vi "PSTR-Initialize Data.vi"(0 "PSTR Params":T1={"Stimulus"={"Ear"=enum."Right", "BW (oct)"=0.25, "Seed"=37, "Ramp (ms)"=5.0, "On time (ms)"=300.0, "Off time (ms)"=300.0, "Delay (ms)"=10000.0}, "FreqSeq"={"Min (kHz)"=4.0, "Max (kHz)"=64.0, "Step (oct)"=0.5}, "LevelSeq"={"Min (dB)"=0.0, "Max (dB)"=80.0, "Step (dB)"=20.0}, "Seq"={"Order"=enum."Sequential", "Averages"=20}, "Response"={"Grass gain"=10000.0, "Window (ms)"=0.0}, "Hidden"={"Sample rate (Hz)"=200000.0, "Nfft"=0, "save raw"=FALSE, "sep"=0.0, "Window"=enum."NONE"}, "RejThr"=0.0}) -> (8 "Data":T10, 15 "error out":errorcluster)   [LabVIEW 2020]
uses:
  Typedefs/PSTR-Data.ctl
  Typedefs/PSTR-Fit Parameters.ctl
  Typedefs/PSTR-Model Fit.ctl
  epl-vi-lib/Utility VIs/Math VIs/LinSpace (x0-dx-npts).vi
  epl-vi-lib/Utility VIs/Math VIs/LinSpace (start-stop-step).vi
  Utility VIs/Type Defs/Left-Right ring.ctl
  Typedefs/PSTR-Stimulus Params.ctl
  Typedefs/PSTR-FreqSeq Params.ctl
  Typedefs/PSTR-LevelSeq Params.ctl
  Typedefs/PSTR-SeqParams.ctl
  Typedefs/PSTR-Response Params.ctl
  Typedefs/PSTR-Hidden Params.ctl
  Typedefs/PSTR-Parameters.ctl
  Typedefs/PSTR-Window Shape.ctl
panel:
  # "NF x NL x 2 x Npts"
  # "NF x NL x Npts"
  # "NF x NL"
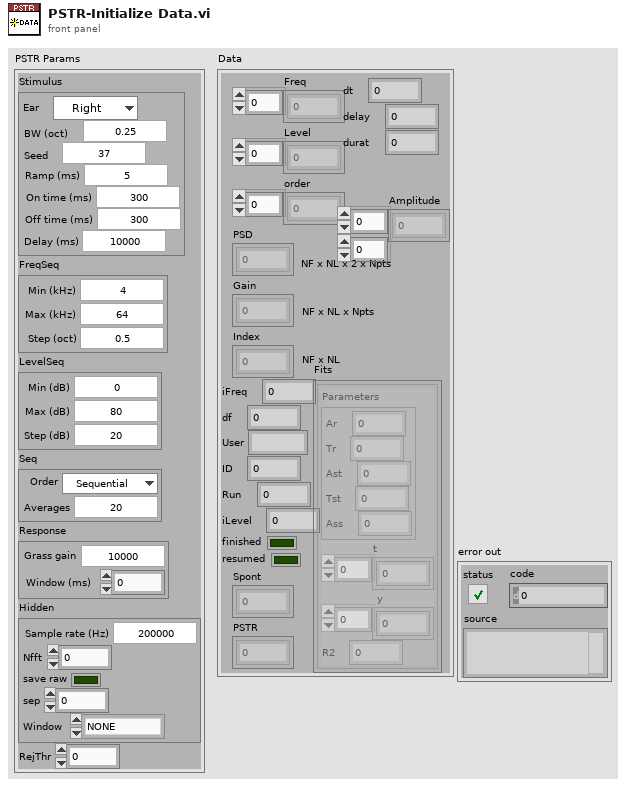
[diagram p1: front panel]
types:
  T1 = typedef "PSTR-Parameters.ctl" = cluster{"Stimulus":T2, "FreqSeq":T4, "LevelSeq":T5, "Seq":T6, "Response":T7, "Hidden":T8, "RejThr":dbl}
  T2 = typedef "PSTR-Stimulus Params.ctl" = cluster{"Ear":T3, "BW (oct)":dbl, "Seed":i32, "Ramp (ms)":dbl, "On time (ms)":dbl, "Off time (ms)":dbl, "Delay (ms)":dbl}
  T3 = typedef "Left-Right ring.ctl" = enum16{"Right", "Left"}
  T4 = typedef "PSTR-FreqSeq Params.ctl" = cluster{"Min (kHz)":dbl, "Max (kHz)":dbl, "Step (oct)":dbl}
  T5 = typedef "PSTR-LevelSeq Params.ctl" = cluster{"Min (dB)":dbl, "Max (dB)":dbl, "Step (dB)":dbl}
  T6 = typedef "PSTR-SeqParams.ctl" = cluster{"Order":enum16{"Sequential", "Random"}, "Averages":i32}
  T7 = typedef "PSTR-Response Params.ctl" = cluster{"Grass gain":dbl, "Window (ms)":dbl}
  T8 = typedef "PSTR-Hidden Params.ctl" = cluster{"Sample rate (Hz)":dbl, "Nfft":i32, "save raw":bool, "sep":dbl, "Window":T9}
  T9 = typedef "PSTR-Window Shape.ctl" = enum16{"NONE", "Hamming"}
  T10 = typedef "PSTR-Data.ctl" = cluster{"Freq":dbl[], "Level":dbl[], "order":i32[], "PSD":dbl[][][][], "Gain":dbl[][][], "Index":dbl[][], "iFreq":i32, "df":dbl, "User":string, "ID":i32, "Run":i32, "iLevel":i32, "finished":bool, "resumed":bool, "Spont":dbl[][], "PSTR":dbl[][][], "dt":dbl, "delay":dbl, "durat":dbl, "Fits":T11[][], "Amplitude":dbl[][]}
  T11 = typedef "PSTR-Model Fit.ctl" = cluster{"Parameters":T12, "t":dbl[], "y":dbl[], "R2":dbl}
  T12 = typedef "PSTR-Fit Parameters.ctl" = cluster{"Ar":dbl, "Tr":dbl, "Ast":dbl, "Tst":dbl, "Ass":dbl}
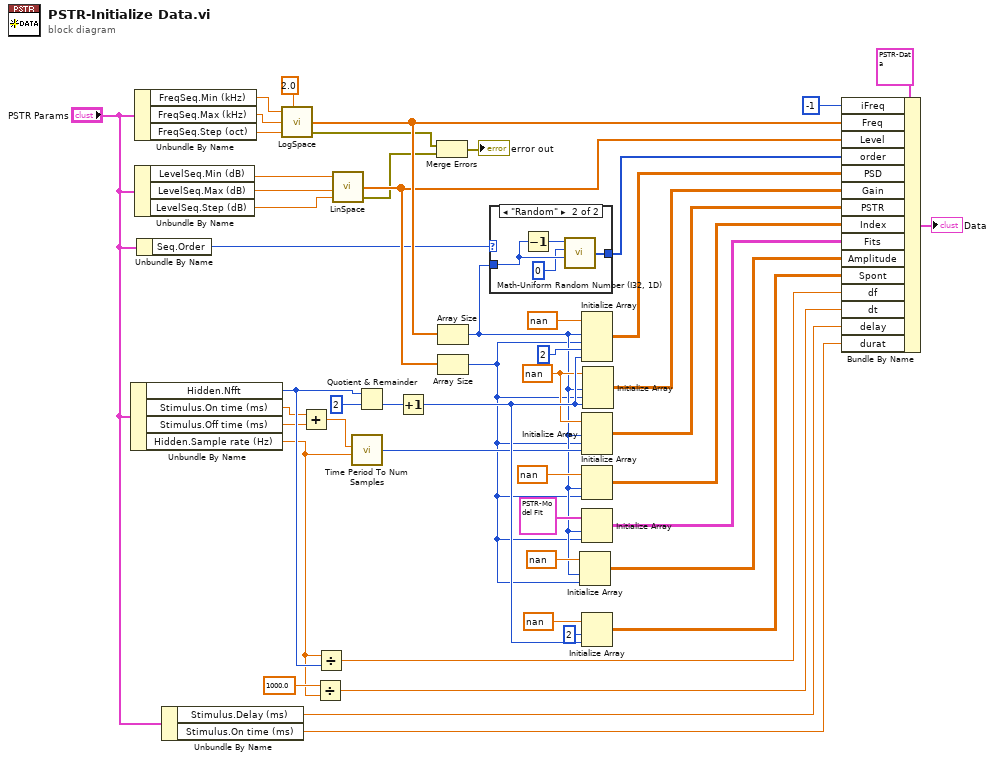
[diagram p0: block diagram]
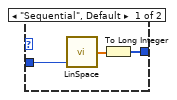
[diagram p2: hidden frame]
diagram:
  w10 = nan ("element")
  n1 = Unbundle By Name("PSTR Params") -> ("Hidden.Nfft"=w25:i32, "Stimulus.On time (ms)"=w14:dbl, "Stimulus.Off time (ms)"=w11:dbl, "Hidden.Sample rate (Hz)"=w13:dbl)
  n2 = Unbundle By Name("PSTR Params") -> ("FreqSeq.Min (kHz)"=w49:dbl, "FreqSeq.Max (kHz)"=w48:dbl, "FreqSeq.Step (oct)"=w47:dbl)
  n3 = Unbundle By Name("PSTR Params") -> ("LevelSeq.Min (dB)"=w42:dbl, "LevelSeq.Max (dB)"=w41:dbl, "LevelSeq.Step (dB)"=w40:dbl)
  n4 = Unbundle By Name("PSTR Params") -> ("Seq.Order"=w29:enum16{"Sequential", "Random"})
  n5 = Unbundle By Name("PSTR Params") -> ("Stimulus.Delay (ms)"=w8:dbl, "Stimulus.On time (ms)"=w7:dbl)
  n6 = call "LogSpace.vi"("Start"=w49, "Base"=2.0, "Stop"=w48, "Step"=w47) -> ("Array"=w38:dbl[], "error out"=w31:errorcluster)  [unwired: 2 in]
  n7 = Add(x=w14, y=w11) -> (x+y=w12:dbl)
  n8 = Divide(x=1000.0, y=w13) -> (x/y=w19:dbl)
  n9 = Divide(x=w13, y=w25) -> (x/y=w20:dbl)
  n10 = call-poly "LinSpace.vi"("Step"=w40, "Stop"=w41, "Start"=w42) -> ("error out"=w30:errorcluster, "Array"=w37:dbl[])  [unwired: 1 in]
  n11 = call "Time Period To Num Samples.vi"("Duration (ms)"=w12, "Sampling rate (Hz)"=w13) -> ("Samples"=w15:i32)  [unwired: 5 in]
  n12 = Quotient & Remainder(x=w25, y=2) -> (floor(x/y)=w26:i32)  [unwired: 1 out]
  n13 = Increment(x=w26) -> (x+1=w18:i32)
  n14 = Merge Errors(w31, w30) -> (→"error out":errorcluster)
  n15 = Array Size(array=w38) -> (size(s)=w3:i32)
  n16 = Array Size(array=w37) -> (size(s)=w2:i32)
  n17 = case shown="\"Random\"" w29 {
    tunnel: w3 -> [w52 w54]
    tunnel: [w50 w55] -> w28
    frame "Sequential", Default {
      n18 = call-poly "LinSpace.vi"("npts"=w52) -> ("Array"=w51:dbl[])  [unwired: 3 in, 1 out]
      n19 = To Long Integer(number=w51) -> (32bit integer=w50:i32[])
    }
    frame "Random" {
      n20 = Decrement(x=w54) -> (x-1=w56:i32)
      n21 = call "Math-Uniform Random Number (I32, 1D).vi"("N"=w54, "Ymin"=0, "Ymax"=w56) -> ("Random Ints"=w55:i32[])  [unwired: 3 in]
    }
  }
  n22 = Initialize Array(nan ("element"), w3, w2) -> (w1:dbl[][])
  n23 = Initialize Array(nan ("element"), w3, w2, 2 ("dimension size"), w18) -> (w35:dbl[][][][])
  n24 = Initialize Array(w10, w3, w2, w15) -> (w16:dbl[][][])
  n25 = Initialize Array(nan ("element"), w3, w2) -> (w33:dbl[][])
  n26 = Initialize Array(T11 {"Parameters"={"Ar"=0.0, "Tr"=0.0, "Ast"=0.0, "Tst"=0.0, "Ass"=0.0}, "t"=[], "y"=[], "R2"=0.0} ("Fit"), w3, w2) -> (w5:T11[][])
  n27 = Initialize Array(nan ("element"), 2 ("dimension size"), w18) -> (w23:dbl[][])
  n28 = Initialize Array(w10, w3, w2, w18) -> (w17:dbl[][][])
  n29 = Bundle By Name(cluster=T10 {"Freq"=[], "Level"=[], "order"=[], "PSD"=[], "Gain"=[], "Index"=[], "iFreq"=0, "df"=0.0, "User"="", "ID"=0, "Run"=0, "iLevel"=0, "finished"=FALSE, "resumed"=FALSE, "Spont"=[], "PSTR"=[], "dt"=0.0, "delay"=0.0, "durat"=0.0, "Fits"=[], "Amplitude"=[]} ("Data"), "iFreq"=-1, "Freq"=w38, "Level"=w37, "order"=w28, "PSD"=w35, "Gain"=w17, "PSTR"=w16, "Index"=w33, "Fits"=w5, "Amplitude"=w1, "Spont"=w23, "df"=w20, "dt"=w19, "delay"=w8, "durat"=w7) -> (→"Data":T10)
